vi "Write Boolean.vi"(8 "error in (no error)":errorcluster, 10 "Boolean":bool, 11 "KDemoBase in":refnum<class "KDemoBase.lvclass">) -> (0 "error out":errorcluster, 3 "KDemoBase out":refnum<class "KDemoBase.lvclass">)   [LabVIEW 2015, in "KDemoBase.lvclass"]
uses:
  KDemoBase.lvclass
  KDemoBase.lvclass/KDemoBase.ctl
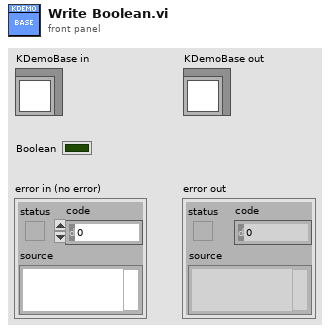
[diagram p1: front panel]
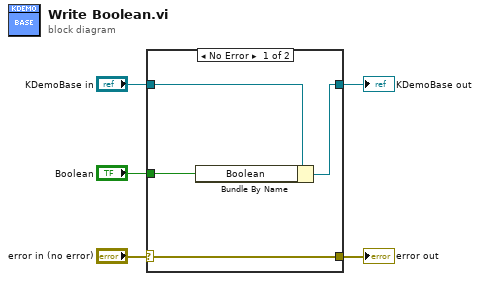
[diagram p0: block diagram]
diagram:
  n1 = case shown="No Error" "error in (no error)" {
    selector: "error in (no error)" -> [w9 w10]
    tunnel: [w9 w10] -> w4
    tunnel: [w7 w11] -> w2
    tunnel: "KDemoBase in" -> [w8 w11]
    tunnel: "Boolean" -> [w6 _]
    frame No Error {
      n2 = Bundle By Name(cluster=w8, "Boolean"=w6) -> (w7:refnum<class "KDemoBase.lvclass">)
    }
    frame Error {
    }
  }
  "error out" <- w4
  "KDemoBase out" <- w2
